vi "Forcing.vi"() -> ()   [LabVIEW 2023]
doc: "Illustrates how to use the NI Scan Engine Forcing VIs to programmatically force values of analog variables."
uses:
  <vilib>/Platform/TimedLoop/XDataNode/timing_clust.ctl
  <vilib>/Platform/TimedLoop/XDataNode/nitl_modes.ctl
  <vilib>/Platform/TimedLoop/XDataNode/wakeup.ctl
  <vilib>/Platform/TimedLoop/XDataNode/XDataNode.xnode
  <vilib>/Platform/TimedLoop/XDataNode/XDNodeRunTimeDep.lvlib
panel:
  in  "Value to Force":dbl
  in  "Forcing Action":enum32{"Force", "Unforce"}(radio)
  in  "Variable Path (URL)":string="\\\\0.0.0.0\\Mod0\\AI0"
  in  "Stop":bool
  out "Forced Output":dbl(graph)
  # "Overview: Use Forcing VIs to programmatically force values of analog variables.\nRequirements: NI-RIO driver\nInstructions:\n1. In Measurement & Automation Explorer, ensure that LabVIEW Real-Time and the NI Scan Engine are installed on your RT target.\n2. From the Project Explorer window, set the IP address of your RT target. \n3. (Optional) You can run this VI on either the host computer or on the RT target.  If you want to run the VI on the RT target, drag Forcing.vi from the My Computer directory to the RT Target directory within the Project Explorer window.\n4. On the front panel, enter the path to an I/O variable of the correct type for the VI in the Variable Path (URL) box. The form of the variable path must be as follows: \\\\<Target URL>\\Module Name\\Variable Name. You can find the exact URL of an I/O variable by placing the variable on the block diagram and pressing <Ctrl-H> to view the context help for the variable node.\n5. Run the VI.\n6. Use the Forcing Action and Value to Force controls to force and unforce I/O values.\n7. Click Stop to stop the VI."
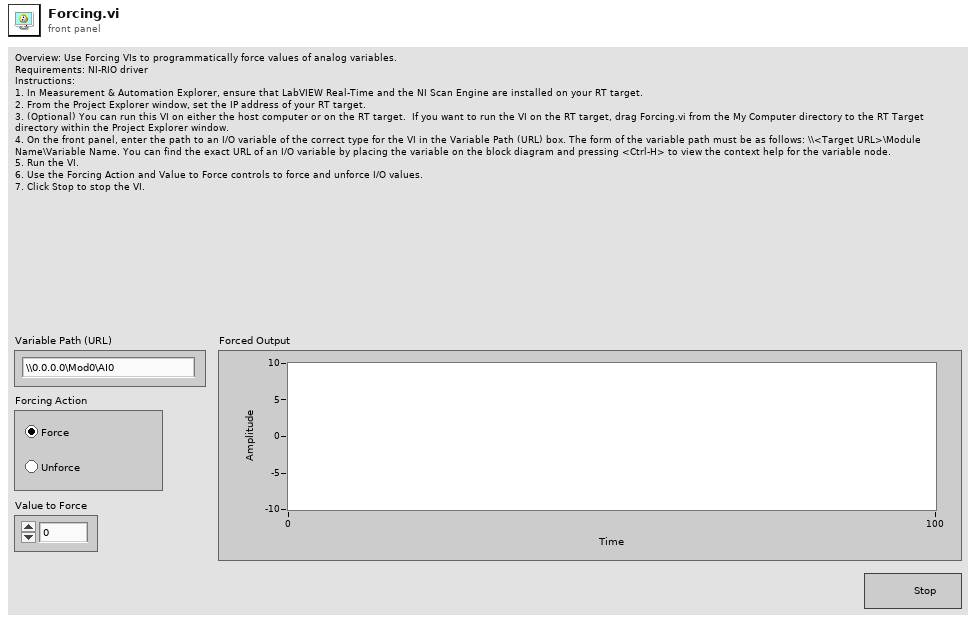
[diagram p1: front panel]
types:
  T1 = typedef "XDNodeRunTimeDep.lvlib/timing_clust.ctl" = cluster{"Expected End [f-1]":u64, "Actual End [f-1]":u64, "Finished Late? [f-1]":bool, "Expected End [i-1]":u64, "Actual End [i-1]":u64, "Finished Late? [i-1]":bool, "Expected Start [i]":u64, "Actual Start [i]":u64, "Expected Start [f]":u64, "Actual Start [f]":u64, "Source Name":string, "Structure Name":string, "Period":i64, "Deadline":i64, "Offset":i64, "Start":i64, "Priority":i32, "Timeout":i32, "Mode":T2, "Wakeup Reason":T3, "Error":errorcluster, "Source Type":string, "Secondary Source Type":string, "Global End Time":u64, "Global Start Time":u64, "Frame Duration":u64, "Iteration Duration":u64, "Assigned CPU":i32, "I/O Scan Engine Mode":u32}
  T2 = typedef "XDNodeRunTimeDep.lvlib/nitl_modes.ctl" = enum32{"No Change", "Process missed periods, maintain original phase", "Discard missed periods, maintain original phase", "Process missed periods, ignore original phase", "Discard missed periods, ignore original phase"}
  T3 = typedef "XDNodeRunTimeDep.lvlib/wakeup.ctl" = enum32{"Normal", "Aborted", "Asynchronous wakeup", "Timing source error", "Timed loop error", "Timeout"}
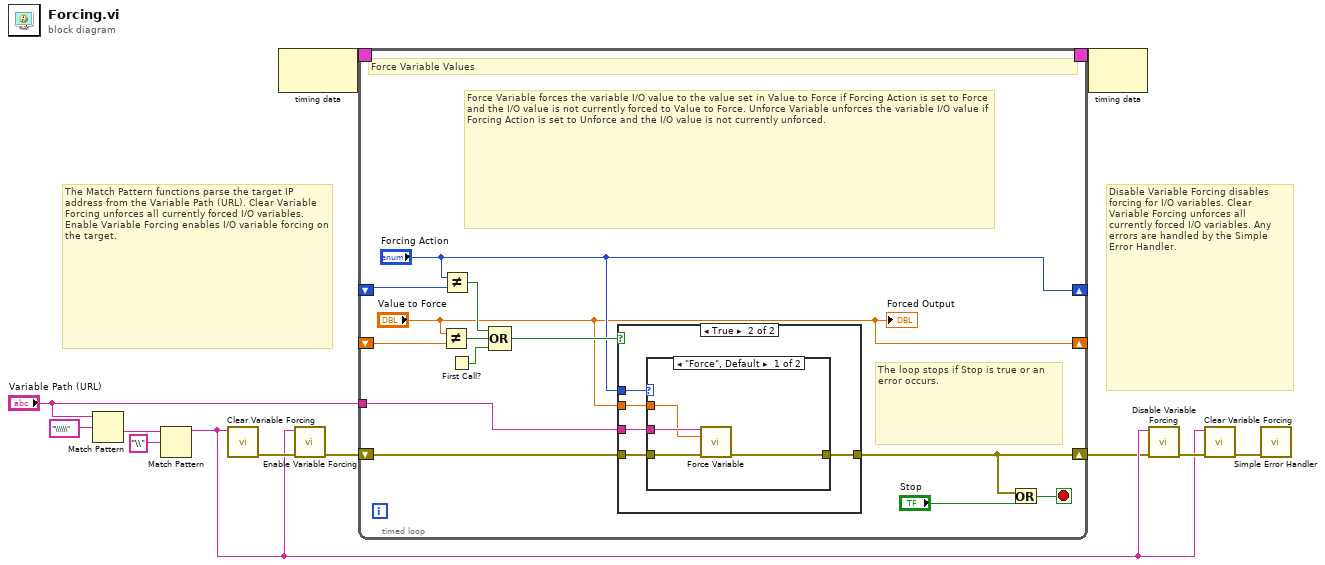
[diagram p0: block diagram]
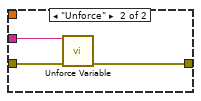
[diagram p3: hidden frame]
diagram:
  # "Disable Variable Forcing disables forcing for I/O variables. Clear Variable Forcing unforces all currently forced I/O variables. Any errors are handled by the Simple Error Handler."
  # "The Match Pattern functions parse the target IP address from the Variable Path (URL). Clear Variable Forcing unforces all currently forced I/O variables. Enable Variable Forcing enables I/O variable forcing on the target."
  n1 = Match Pattern(string="Variable Path (URL)", regular expression="\\\\\\") -> (after substring=w8:string)  [unwired: 4 out]
  n2 = Match Pattern(string=w8, regular expression="\\") -> (before substring=w4:string)  [unwired: 4 out]
  n3 = call <vilib>:"Clear Variable Forcing.vi"("target address (localhost)"=w4) -> ("error out"=w6:errorcluster)  [unwired: 1 in, 7 out]
  n4 = node-c288() -> (w12:T1)  [unwired: 1 out]
  n5 = call <vilib>:"Enable Variable Forcing.vi"("error in (no error)"=w6, "target address (localhost)"=w4) -> ("error out"=w2:errorcluster)  [unwired: 7 out]
  n6 = timed-loop {
    shift-right: ["Value to Force"] -> _
    shift-left: _ -> [w23]
    shift-right: ["Forcing Action"] -> _
    shift-left: _ -> [w22]
    timing: w12 -> [_]
    timing-out: [_] -> w11
    tunnel: "Variable Path (URL)" -> [w15]
    shift-right: [w13] -> w1
    shift-left: w2 -> [w14]
    stop <- w24 stop-if-true
    # "Force Variable forces the variable I/O value to the value set in Value to Force if Forcing Action is set to Force and the I/O value is not currently forced to Value to Force. Unforce Variable unforces the variable I/O value if Forcing Action is set to Unforce and the I/O value is not currently unforced."
    # "The loop stops if Stop is true or an error occurs."
    # "Force Variable Values"
    n7 = Not Equal?(x="Value to Force", y=w23) -> (x != y?=w19:bool)
    n8 = Not Equal?(x="Forcing Action", y=w22) -> (x != y?=w20:bool)
    n9 = First Call?() -> (First Call?: T/F=w21:bool)
    n10 = Compound Arithmetic op=OR(w20, w19, w21) -> (w18:bool)
    n11 = case shown="True" w18 {
      tunnel: w14 -> [w26 w31]
      tunnel: w15 -> [_ w30]
      tunnel: [w26 w29] -> w13
      tunnel: "Forcing Action" -> [_ w28]
      tunnel: "Value to Force" -> [_ w27]
      frame False {
      }
      frame True {
        n12 = case shown="\"Force\", Default" w28 {
          tunnel: w31 -> [w35 w38]
          tunnel: w30 -> [w34 w36]
          tunnel: [w33 w37] -> w29
          tunnel: w27 -> [w32 _]
          frame "Force", Default {
            n13 = call <vilib>:"Force Variable.vi"("variable path (URL)"=w34, "forced value"=w32, "error in (no error)"=w35) -> ("error out"=w33:errorcluster)  [unwired: 12 out]
          }
          frame "Unforce" {
            n14 = call <vilib>:"Unforce Variable.vi"("variable path (URL)"=w36, "error in (no error)"=w38) -> ("error out"=w37:errorcluster)  [unwired: 13 out]
          }
        }
      }
    }
    n15 = Or(x=w13, y="Stop") -> (x .or. y?=w24:bool)
    "Forced Output" <- "Value to Force"
  }
  n16 = node-c288(w11) -> ()  [unwired: 1 out]
  n17 = call <vilib>:"Disable Variable Forcing.vi"("error in (no error)"=w1, "target address (localhost)"=w4) -> ("error out"=w5:errorcluster)  [unwired: 7 out]
  n18 = call <vilib>:"Clear Variable Forcing.vi"("error in (no error)"=w5, "target address (localhost)"=w4) -> ("error out"=w3:errorcluster)  [unwired: 7 out]
  n19 = call <vilib>:"Simple Error Handler.vi"("error in (no error)"=w3) -> ()  [unwired: 1 in, 8 out]
